vi "MakeSuperLink.vi"(11 "data":string) -> (1 "show info":string, 2 "superlinkStr":string, 3 "Accept":bool)   [LabVIEW 2011, in "XSuperLink.xctl"]
uses:
  XSuperLink.xctl
  <vilib>/regexp/Match Regular Expression.xnode
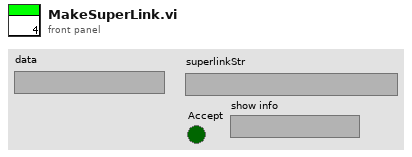
[diagram p1: front panel]
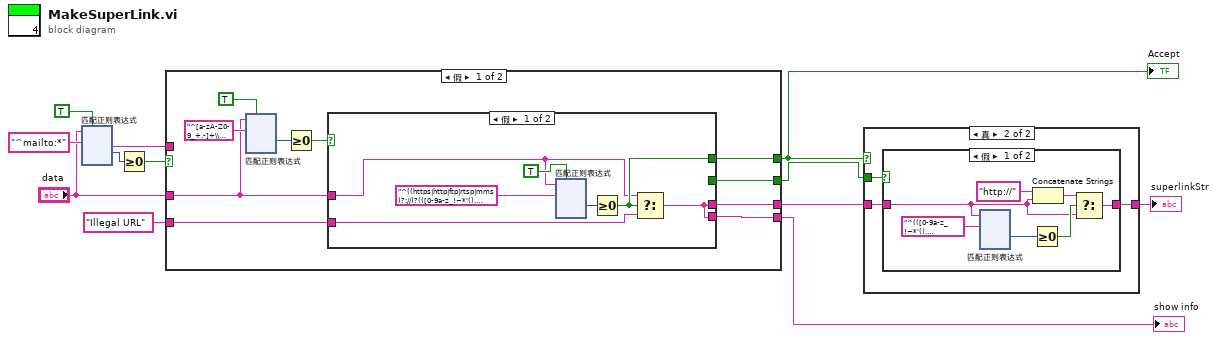
[diagram p0: block diagram]
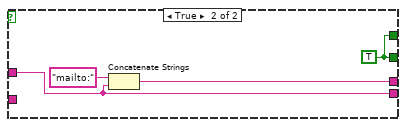
[diagram p4: hidden frame]
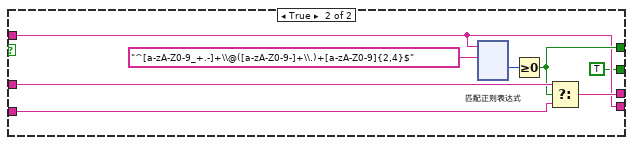
[diagram p5: hidden frame]
diagram:
  n1 = xnode "匹配正则表达式"("输入字符串"="data", "正则表达式"="^mailto:*", "忽略大小写？(F)"=TRUE) -> ("匹配之后"=w8:string, "匹配后偏移量"=w10:i32)  [unwired: 3 in, 3 out]
  n2 = Greater Or Equal To 0?(x=w10) -> (x >= 0?=w9:bool)
  n3 = case shown="假" w9 {
    tunnel: w8 -> [_ w257]
    tunnel: "data" -> [w18 w261]
    tunnel: [w17 w260] -> w3
    tunnel: [w16 w259] -> w4
    tunnel: "Illegal URL" ("f") -> [w15 w258]
    tunnel: [w14 w257] -> w5
    tunnel: [w13 TRUE] -> w2
    frame False {
      n4 = xnode "匹配正则表达式"("输入字符串"=w18, "正则表达式"="^[a-zA-Z0-9_+.-]+\\@([a-zA-Z0-9-]+\\.)+[a-zA-Z0-9]{2,4}$", "忽略大小写？(F)"=TRUE) -> ("匹配后偏移量"=w20:i32)  [unwired: 3 in, 4 out]
      n5 = Greater Or Equal To 0?(x=w20) -> (x >= 0?=w19:bool)
      n6 = case shown="假" w19 {
        tunnel: w18 -> [w25 w142]
        tunnel: [w23 w143] -> w17
        tunnel: [w26 w141] -> w16
        tunnel: w15 -> [w24 _]
        tunnel: [w23 w142] -> w14
        tunnel: [_ w141] -> w13
        frame False {
          n7 = xnode "匹配正则表达式"("输入字符串"=w25, "正则表达式"="^((https|http|ftp|rtsp|mms)?://)?(([0-9a-z_!~*'().&=+$%-]+: )?[0-9a-z_!~*'().&=+$%-]+@)?(([0-9]{1,3}\\.){3}[0-9]{1,3}|([0-9a-z_!~*'()-]+\\.)*([0-9a-z][0-9a-z-]{0,61})?[0-9a-z]\\.[a-z]{2,6})(:[0-9]{1,4})?((/?)|(/[0-9a-z_!~*'().;?:@&=+$,%#-]+)+/?)$", "忽略大小写？(F)"=TRUE) -> ("匹配后偏移量"=w27:i32)  [unwired: 3 in, 4 out]
          n8 = Greater Or Equal To 0?(x=w27) -> (x >= 0?=w26:bool)
          n9 = Select(t=w25, s=w26, f=w24) -> (s? t:f=w23:string)
        }
        frame True {
          w141 = TRUE
          n10 = Concatenate Strings("mailto:" ("字符串"), w142) -> (w143:string)
        }
      }
    }
    frame True {
      n11 = xnode "匹配正则表达式"("输入字符串"=w257, "正则表达式"="^[a-zA-Z0-9_+.-]+\\@([a-zA-Z0-9-]+\\.)+[a-zA-Z0-9]{2,4}$") -> ("匹配后偏移量"=w262:i32)  [unwired: 4 in, 4 out]
      n12 = Greater Or Equal To 0?(x=w262) -> (x >= 0?=w259:bool)
      n13 = Select(t=w261, s=w259, f=w258) -> (s? t:f=w260:string)
    }
  }
  "Accept" <- w4
  "show info" <- w5
  n14 = case shown="真" w4 {
    tunnel: w3 -> [w375 w377]
    tunnel: w2 -> [_ w378]
    tunnel: [w375 w376] -> w1
    frame False {
    }
    frame True {
      n15 = case shown="假" w378 {
        tunnel: w377 -> [w380 w497]
        tunnel: [w379 w497] -> w376
        frame False {
          n16 = xnode "匹配正则表达式"("输入字符串"=w380, "正则表达式"="^(([0-9a-z_!~*'().&=+$%-]+: )?[0-9a-z_!~*'().&=+$%-]+@)?(([0-9]{1,3}\\.){3}[0-9]{1,3}|([0-9a-z_!~*'()-]+\\.)*([0-9a-z][0-9a-z-]{0,61})?[0-9a-z]\\.[a-z]{2,6})(:[0-9]{1,4})?((/?)|(/[0-9a-z_!~*'().;?:@&=+$,%#-]+)+/?)$") -> ("匹配后偏移量"=w384:i32)  [unwired: 4 in, 4 out]
          n17 = Greater Or Equal To 0?(x=w384) -> (x >= 0?=w383:bool)
          n18 = Concatenate Strings("http://" ("字符串"), w380) -> (w381:string)
          n19 = Select(t=w381, s=w383, f=w380) -> (s? t:f=w379:string)
        }
        frame True {
        }
      }
    }
  }
  "superlinkStr" <- w1
